vi "_PC_Daemon_SaveFiles.vi"(7 "SigProc.Enable":bool caption="SigProc", 8 "error in (no error)":errorcluster, 11 "Document Path":path) -> (0 "error out":errorcluster)   [LabVIEW 2018]
uses:
  RecipeEditorPython/subVI/getScriptInfo.ctl
  RT/PublicSubVI/Ctl/_ctl_RT_ExpCondi.ctl
  SaveFile/DataTree/ctl/FMstateMachineEnum.ctl
  PublicSubVI/Class/FileManager/FM/ctl/_PC_Pub_FM ctrlFileRefnumEnum.ctl
  PublicSubVI/Ctl/RegistyFunc.ctl
  <vilib>/Utility/miscctls.llb/LVRowAndColumnTypeDef.ctl
  <vilib>/event_ctls.llb/eventvkey.ctl
  PublicSubVI/Overload/Experiment Condition/_PC_Pub_ExpCondiValue_Script.vi
  PublicSubVI/Class/QMH/QMH.lvclass
  SaveFile/DataTree/DataTreeCtrl.lvclass
  PublicSubVI/Class/Sig2MS/Sig2MS.lvclass
panel:
  in  "Tab Control":enum32{"Document", "File"}(tab)
  in  "Document Tree":string[](tree)=["D:\\ATI_MS_InstrumentControl_08_08_15\\MSData\\Test\\Untitled.flist"]
  in  "Undo":bool
  in  "File Tree":string[](tree)
  out "wfmGraph":waveform(sgl)[](graph)
  out "XY Graph":cluster{"X":dbl[], "Y":sgl[]}[](graph)
  in  "listDataInfo":i32(listbox)=-1
  out "Item Names":string[](array[string])
  in  "mouse state":T1(ring)
  in  "timeDomain":bool caption="Time Domain"
  in  "Cursor":bool
  out "Y :":dbl
  out "X :":dbl
  in  "MergePlots":bool
  in  "SigProc.Edit":bool
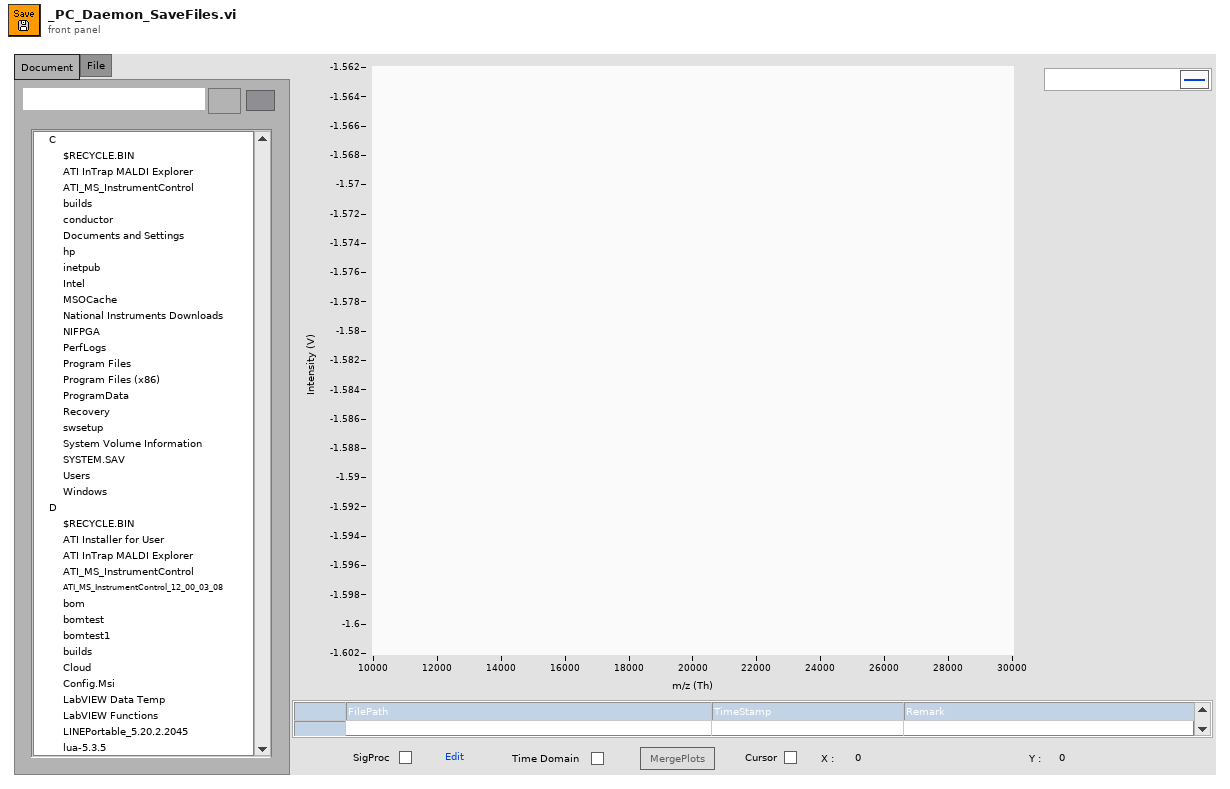
[diagram p1: front panel]
types:
  T1 = enum16{"normal", "select noise", "select signal", "return"}
  T2 = cluster{"xyGraph":refnum<vi>, "wfmGraph":refnum<vi>, "docPath in":refnum<vi>}
  T3 = enum8{"Enabled", "Disabled", "Disabled and Grayed Out"}
  T4 = cluster{"xyGraph":refnum<vi>, "wfmGraph":refnum<vi>}
  T5 = typedef "getScriptInfo.ctl" = enum16{"userEditor", "userParam", "instrParam", "sourcePath", "sourceTimeStamp", "versionInfo"}
  T6 = typedef "_ctl_RT_ExpCondi.ctl" = cluster{"Label":string, "Value":variant}[]
  T7 = cluster{"selectDataArr":string[], "tagFilePath":string}
  T8 = typedef "FMstateMachineEnum.ctl" = enum16{"none", "init", "openTDMS", "closeTDMS", "getDataList", "getDataInfo", "getTimeStamp", "getCurrPath", "getRemark", "overwriteRemark", "readData", "deleteData", "moveData"}
  T9 = typedef "_PC_Pub_FM ctrlFileRefnumEnum.ctl" = enum16{"init", "checkFileName", "updFileName", "updWorkFolder", "updDataItems", "addNewFileName", "addSerialNum"}
  T10 = cluster{"xyXLabel":string, "xyYLabel":string, "wfmXLabel":string, "wfmYLabel":string}
  T11 = cluster{"dt":dbl, "xdata":dbl[], "ydata":sgl[], "beta":dbl[]}[][]
  T12 = cluster{"startTime":dbl, "scanData":cluster{"dt":dbl, "xdata":dbl[], "ydata":sgl[], "beta":dbl[]}[], "xyXLabel":string, "xyYLabel":string, "wfmXLabel":string, "wfmYLabel":string, "ionData":cluster{"dt":dbl, "ydata":sgl[]}[], "ionXLabel":string, "ionYLabel":string}
  T13 = typedef "RegistyFunc.ctl" = enum16{"None", "FileAutoSave", "FileNoise", "FileSN", "ExeStatu", "WorkFolderPath", "MethodPath", "AVGItem", "LoopItem", "AutoRun", "BGColor", "LineColor", "LineWidth", "XGrid", "YGrid", "DeviceRefnum"}
  T14 = enum16{"init", "loadScript", "newScript", "runScript", "close"}
  T15 = typedef "LVRowAndColumnTypeDef.ctl" = cluster{"Row":i32, "Column":i32}
  T16 = typedef "eventvkey.ctl" = enum16{"ASCII", "Enter", "Return", "Shift", "Ctrl", "Alt", "Cmd", "Opt", "Caps", "NumLock", "Clear", "Break", "Up", "Down", "Left", "Right", "Insert", "Delete", "Home", "End", "PageUp", "PageDown", "Escape", "Help", "Pause", "ScrollLock", "F1", "F2", "F3", "F4", "F5", "F6", "F7", "F8", "F9", "F10", "F11", "F12", "F13", "F14", "F15", "F16", "F17", "F18", "F19", "F20", "F21", "F22", "F23", "F24", "Play", "VolumeUp", "VolumeDown", "Mute", "Two Byte Char"}
  T17 = typedef "LVPoint32TypeDef.ctl" = cluster{"Horizontal":i32, "Vertical":i32}
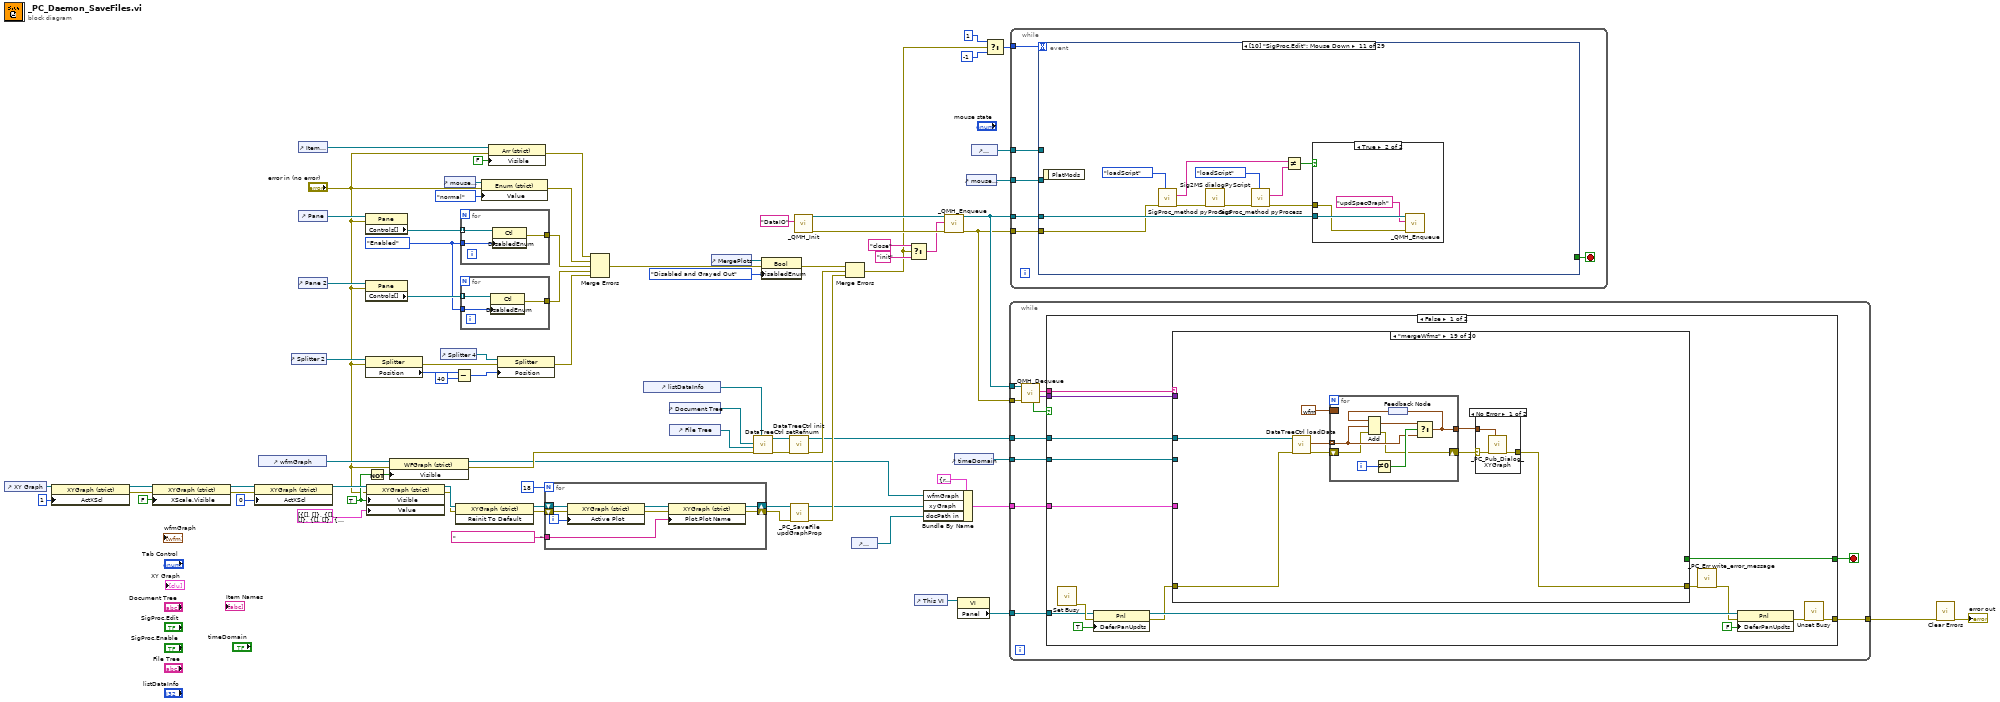
[diagram p0: block diagram]
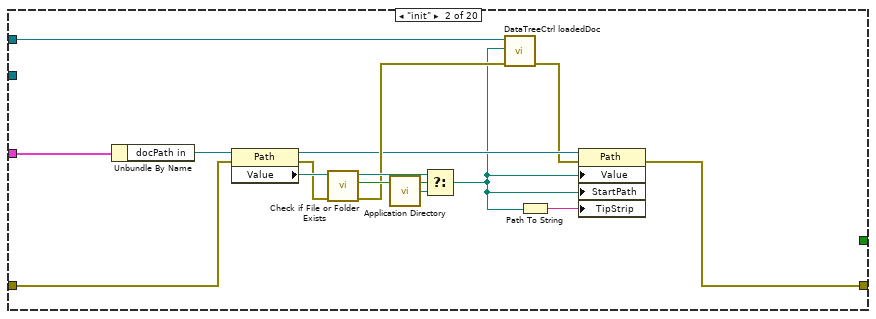
[diagram p3: hidden frame]
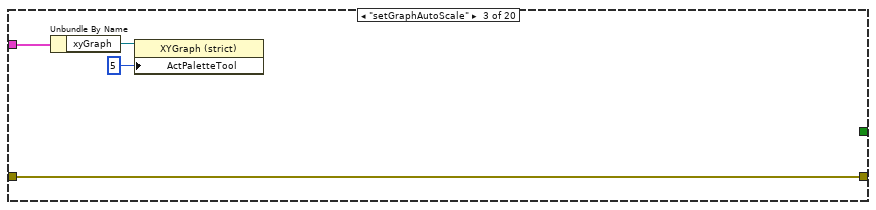
[diagram p4: hidden frame]
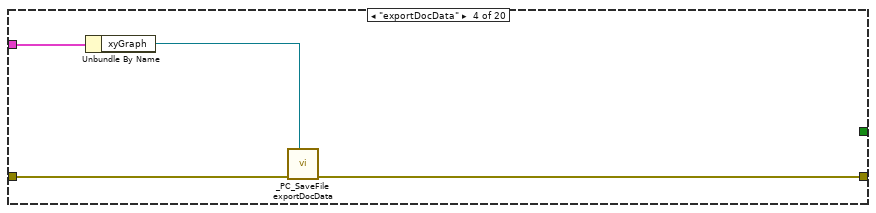
[diagram p5: hidden frame]
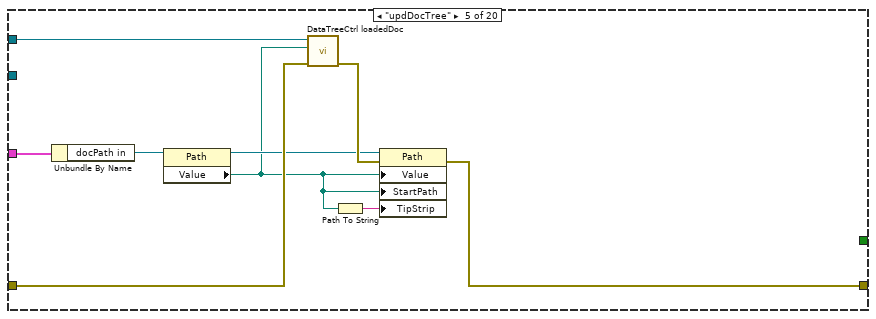
[diagram p6: hidden frame]
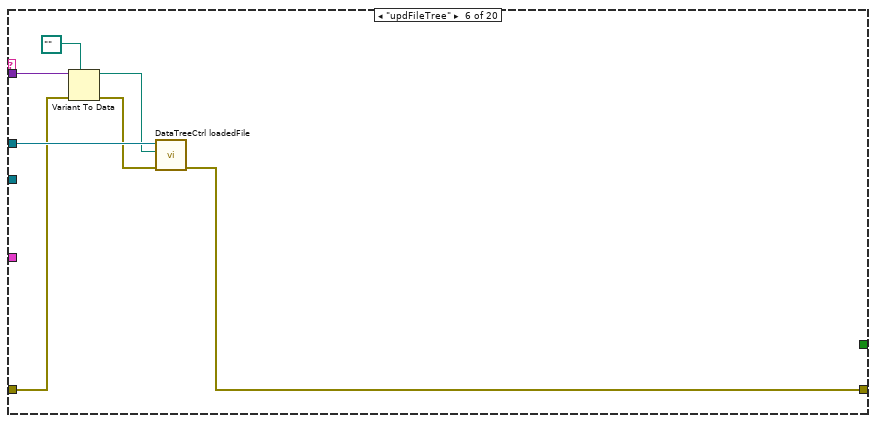
[diagram p7: hidden frame]
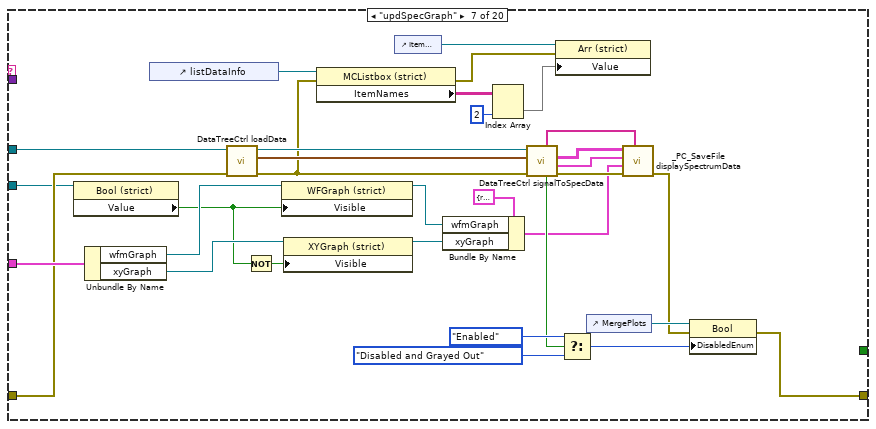
[diagram p8: hidden frame]
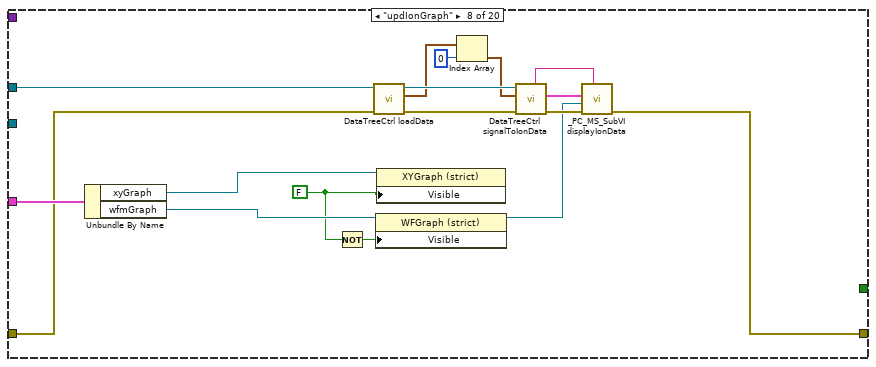
[diagram p9: hidden frame]
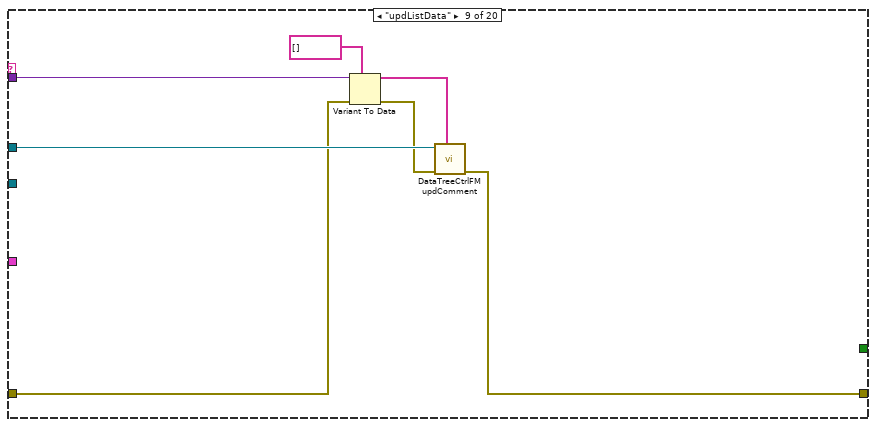
[diagram p10: hidden frame]
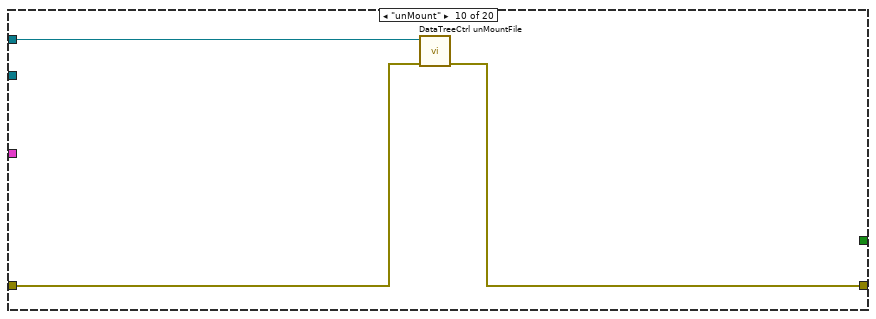
[diagram p11: hidden frame]
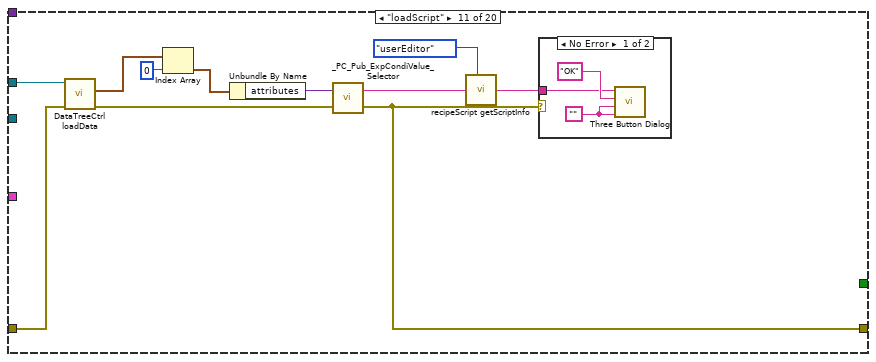
[diagram p12: hidden frame]
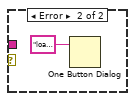
[diagram p13: hidden frame]
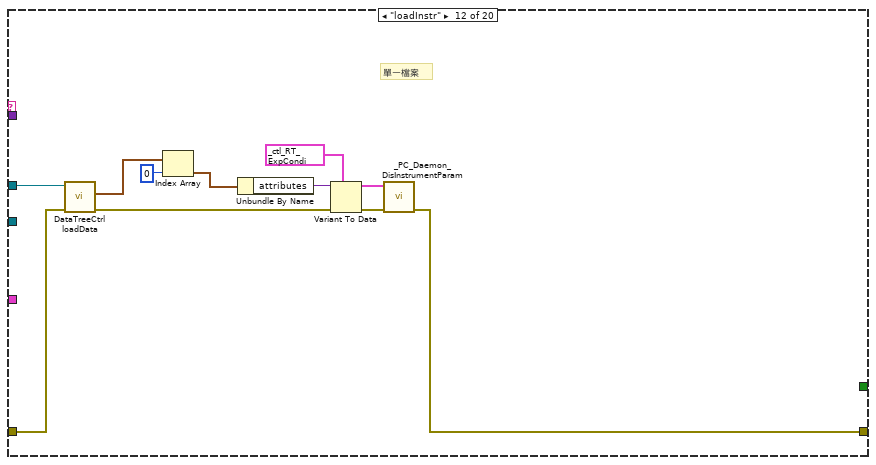
[diagram p14: hidden frame]
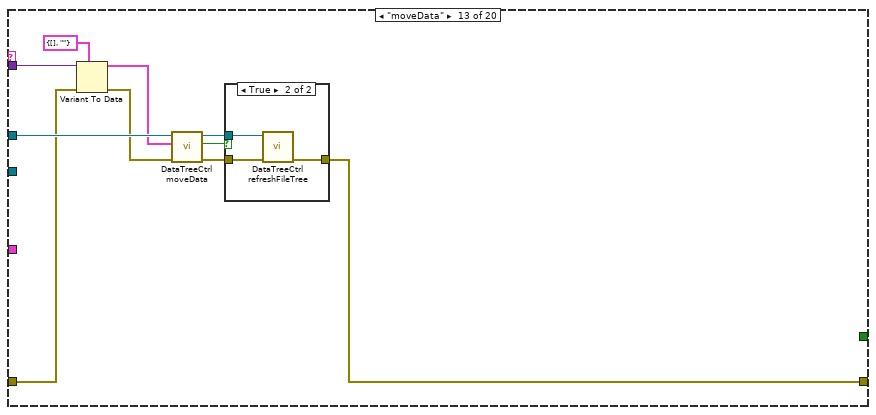
[diagram p15: hidden frame]
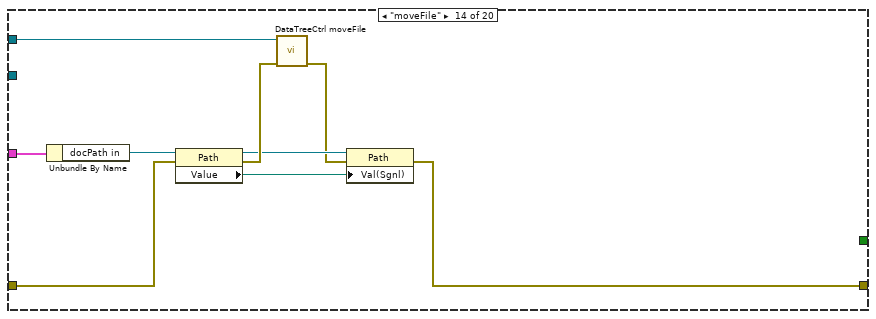
[diagram p17: hidden frame]
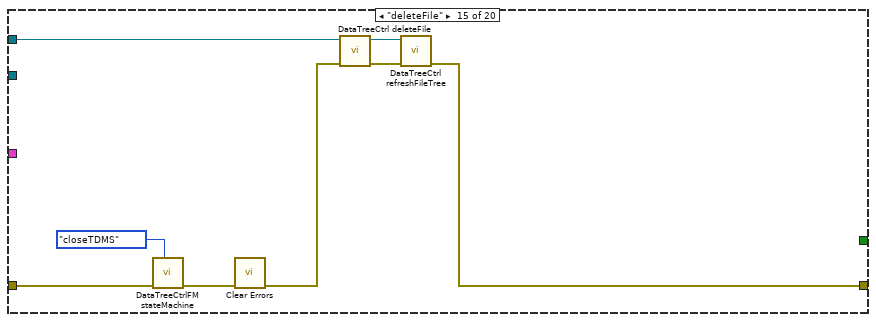
[diagram p18: hidden frame]
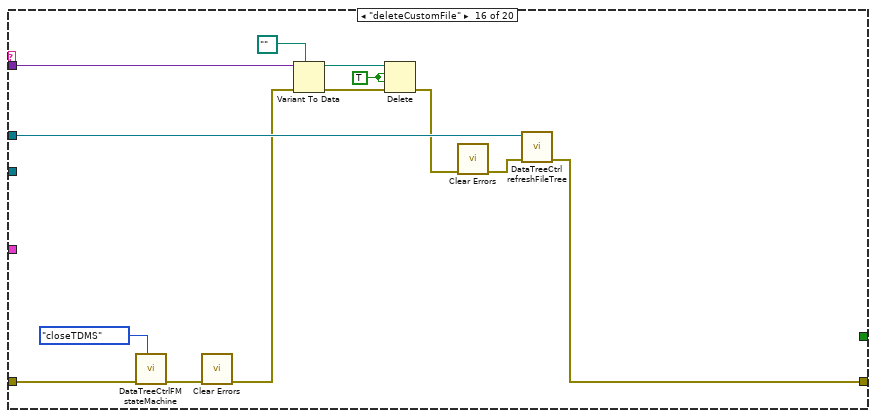
[diagram p19: hidden frame]
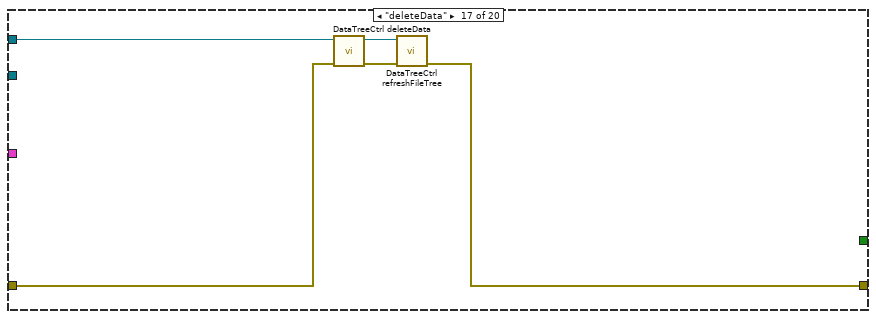
[diagram p20: hidden frame]
diagram:
  w23 = TRUE ("Visible")
  w66 = T3."Enabled" ("Disabled")
  n1 = control-ref of="XY Graph"() -> (w30:refnum<vi>)
  n2 = property class="XYGraph (strict)"(reference=w30, "ActXScl"=1 ("Active X Scale")) -> (reference out=w33:refnum<vi>, error out=w34:errorcluster)  [unwired: 1 in]
  n3 = property class="XYGraph (strict)"(reference=w33, error in=w34, "XScale.Visible"=FALSE ("X Scale.Visible")) -> (reference out=w29:refnum<vi>, error out=w28:errorcluster)
  n4 = property class="XYGraph (strict)"(reference=w29, error in=w28, "ActXScl"=0 ("Active X Scale")) -> (reference out=w26:refnum<vi>)  [unwired: 1 out]
  n5 = control-ref of="wfmGraph"() -> (w24:refnum<vi>)
  n6 = control-ref of="Splitter 2"() -> (w10:refnum<vi>)
  n7 = control-ref of="Item Names"() -> (w13:refnum<vi>)
  n8 = control-ref of="Pane"() -> (w65:refnum<vi>)
  n9 = control-ref of="Pane 2"() -> (w64:refnum<vi>)
  n10 = property class="Pane"(reference=w65, error in="error in (no error)") -> ("Controls[]"=w68:refnum<vi>[])  [unwired: 2 out]
  n11 = property class="Pane"(reference=w64, error in="error in (no error)") -> ("Controls[]"=w67:refnum<vi>[])  [unwired: 2 out]
  n12 = property class="Splitter"(reference=w10, error in="error in (no error)") -> (error out=w5:errorcluster, "Position"=w8:i32)  [unwired: 1 out]
  n13 = property class="XYGraph (strict)"(reference=w26, error in="error in (no error)", "Visible"=w23, "Value"=cluster{dbl[], sgl[]}[] [{[], []}, {[], []}, {[], []}, {[], []}, {[], []}, {[], []}, {[], []}, {[], []}, {[], []}, {[], []}, {[], []}, {[], []}, {[], []}, {[], []}, {[], []}, {[], []}, {[], []}, {[], []}] ("massSpec")) -> (reference out=w59:refnum<vi>, error out=w58:errorcluster)
  n14 = Not(x=w23) -> (.not. x?=w22:bool)
  n15 = property class="WFGraph (strict)"(reference=w24, error in="error in (no error)", "Visible"=w22) -> (reference out=w20:refnum<vi>, error out=w25:errorcluster)
  n16 = control-ref of="Splitter 4"() -> (w9:refnum<vi>)
  n17 = control-ref of="mouse state"() -> (w61:refnum<vi>)
  n18 = Subtract(x=w8, y=40) -> (x-y=w6:i32)
  n19 = invoke class="XYGraph (strict)" method="Reinit To Default"(reference=w59, error in=w58) -> (reference out=w77:refnum<vi>, error out=w52:errorcluster)  [unwired: 1 in, 1 out]
  n20 = for {
    tunnel: w68 -> [w82] mode=indexing
    tunnel: w66 -> [w81]
    tunnel: [w80] -> w63
    n21 = property class="Ctl"(reference=w82, "DisabledEnum"=w81) -> (error out=w80:errorcluster)  [unwired: 1 in, 1 out]
  }
  n22 = for {
    tunnel: w67 -> [w85] mode=indexing
    tunnel: w66 -> [w84]
    tunnel: [w83] -> w62
    n23 = property class="Ctl"(reference=w85, "DisabledEnum"=w84) -> (error out=w83:errorcluster)  [unwired: 1 in, 1 out]
  }
  n24 = property class="Enum (strict)"(reference=w61, error in="error in (no error)", "Value"=T1."normal") -> (error out=w60:errorcluster)  [unwired: 1 out]
  n25 = property class="Arr (strict)"(reference=w13, error in="error in (no error)", "Visible"=FALSE) -> (error out=w11:errorcluster)  [unwired: 1 out]
  n26 = property class="Splitter"(reference=w9, error in=w5, "Position"=w6) -> (error out=w3:errorcluster)  [unwired: 1 out]
  n27 = for {
    N: 18 -> [_]
    tunnel: "                                          " -> [w91]
    shift-right: [w86] -> w51
    shift-left: w52 -> [w87]
    shift-right: [w88] -> w72
    shift-left: w77 -> [w93]
    i -> [w92]
    n28 = property class="XYGraph (strict)"(reference=w93, error in=w87, "Active Plot"=w92) -> (reference out=w90:refnum<vi>, error out=w89:errorcluster)
    n29 = property class="XYGraph (strict)"(reference=w90, error in=w89, "Plot.Plot Name"=w91) -> (reference out=w88:refnum<vi>, error out=w86:errorcluster)
  }
  n30 = Merge Errors(w11, w60, w63, w62, w3) -> (w2:errorcluster)
  n31 = control-ref of="listDataInfo"() -> (w14:refnum<vi>)
  n32 = control-ref of="Document Tree"() -> (w56:refnum<vi>)
  n33 = control-ref of="File Tree"() -> (w55:refnum<vi>)
  n34 = control-ref of="MergePlots"() -> (w71:refnum<vi>)
  n35 = call "DataTreeCtrl setRefnum.vi"("listDataInfo"=w14, "error in (no error)"=w25, "File Tree"=w55, "Document Tree"=w56) -> ("error out"=w53:errorcluster, "DataTreeCtrl out"=w54:refnum<class "DataTreeCtrl.lvclass">)  [unwired: 6 in]
  n36 = property class="Bool"(reference=w71, error in=w2, "DisabledEnum"=T3."Disabled and Grayed Out" ("Disabled")) -> (error out=w50:errorcluster)  [unwired: 1 out]
  n37 = call "DataTreeCtrl init.vi"("error in (no error)"=w53, "DataTreeCtrl in"=w54) -> ("error out"=w49:errorcluster, "DataTreeCtrl out"=w41:refnum<class "DataTreeCtrl.lvclass">)  [unwired: 8 in]
  n38 = call "_PC_SaveFile updGraphProp.vi"("error in (no error)"=w51, "XY Graph in"=w72) -> ("error out"=w48:errorcluster, "XY Graph out"=w44:refnum<vi>)  [unwired: 8 in]
  n39 = call "_QMH_Init.vi"("name (unnamed)"="DataIO") -> ("error out"=w73:errorcluster, "QMH out"=w74:refnum<class "QMH.lvclass">)  [unwired: 9 in]
  n40 = Merge Errors(w50, w49, w48) -> (w1:errorcluster)
  n41 = control-ref of="Document Path"() -> (w43:refnum<vi>)
  n42 = Select(t="close" ("Msg"), s=w1, f="init" ("Msg")) -> (s? t:f=w45:string)
  n43 = control-ref of="This VI"() -> (w78:refnum<vi>)
  n44 = Bundle By Name(cluster=T2 {"xyGraph"=refnum, "wfmGraph"=refnum, "docPath in"=refnum}, "wfmGraph"=w20, "xyGraph"=w44, "docPath in"=w43) -> (w42:T2)
  n45 = call "_QMH_Enqueue.vi"("error in (no error)"=w73, "Msg"=w45, "QMH in"=w74) -> ("error out"=w39:errorcluster, "QMH out"=w40:refnum<class "QMH.lvclass">)  [unwired: 7 in]
  n46 = control-ref of="timeDomain"() -> (w19:refnum<vi>)
  n47 = property class="VI"(reference=w78) -> ("Panel"=w38:refnum<vi>)  [unwired: 1 in, 2 out]
  n48 = control-ref of="mouse state"() -> (w69:refnum<vi>)
  n49 = control-ref of="Document Path"() -> (w37:refnum<vi>)
  n50 = Select(t=1, s=w1, f=-1) -> (s? t:f=w15:i32)
  n51 = while {
    tunnel: w42 -> [w98]
    tunnel: w41 -> [w97]
    tunnel: w40 -> [w104]
    tunnel: w39 -> [w103]
    tunnel: w38 -> [w99]
    tunnel: [w95] -> w36
    tunnel: w19 -> [w94]
    stop <- w96 stop-if-true
    n52 = call "_QMH_Dequeue.vi"("error in (no error)"=w103, "QMH in"=w104) -> ("Data"=w100:variant, "Msg"=w101:string, "timed out?"=w102:bool)  [unwired: 4 in, 3 out]
    n53 = case shown="False" w102 {
      tunnel: w101 -> [w120 _]
      tunnel: w100 -> [w119 _]
      tunnel: w99 -> [w116 _]
      tunnel: w98 -> [w109 _]
      tunnel: w97 -> [w108 _]
      tunnel: [w107 _] -> w96
      tunnel: [w106 _] -> w95
      tunnel: w94 -> [w105 _]
      frame False {
        n54 = call <vilib>:"Set Busy.vi"() -> ("error out"=w117:errorcluster)  [unwired: 10 in, 1 out]
        n55 = property class="Pnl"(reference=w116, error in=w117, "DeferPanUpdts"=TRUE ("Defer Panel Updates")) -> (reference out=w113:refnum<vi>, error out=w110:errorcluster)
        n56 = case shown="\"mergeWfms\"" w120 {
          tunnel: w119 -> [_ _ _ _ _ w159 _ _ w214 _ _ _ w251 _ _ w288 _ _ _ _]
          tunnel: [w121 w134 w137 w141 w145 w154 w186 w199 w215 w217 w224 w235 w246 w260 w271 w289 w290 w295 w300 w322] -> w111
          tunnel: w110 -> [w121 w122 w137 w142 w148 w156 w182 w207 w212 w218 w223 w241 w248 w265 w272 w279 w293 w296 w304 w319]
          tunnel: w109 -> [_ w135 w139 w144 w152 _ w192 w209 _ _ _ _ _ w267 _ _ _ _ _ _]
          tunnel: w108 -> [_ w136 _ _ w153 w160 w191 w208 w216 w219 w230 w245 w252 w268 w276 w283 w294 w297 w305 _]
          tunnel: [_ _ _ _ _ _ _ _ _ _ _ _ _ _ _ _ _ _ _ TRUE] -> w107
          tunnel: w105 -> [_ _ _ _ _ _ w176 _ _ _ _ _ _ _ _ _ _ _ _ _]
          frame Default {
          }
          frame "init" {
            n57 = Unbundle By Name(w135) -> ("docPath in"=w130:refnum<vi>)
            n58 = property class="Path"(reference=w130, error in=w122) -> (reference out=w126:refnum<vi>, error out=w128:errorcluster, "Value"=w129:path)
            n59 = call <vilib>:"Check if File or Folder Exists.vi"("error in (no error)"=w128, "path"=w129) -> ("error out"=w127:errorcluster, "file or folder exists?"=w133:bool, "dup path"=w132:path)  [unwired: 7 in]
            n60 = call <vilib>:"Application Directory.vi"() -> ("Application Directory"=w131:path)
            n61 = Select(t=w132, s=w133, f=w131) -> (s? t:f=w125:path)
            n62 = call "DataTreeCtrl loadedDoc.vi"("error in (no error)"=w127, "RootPath"=w125, "DataTreeCtrl in"=w136) -> ("error out"=w123:errorcluster)  [unwired: 7 in, 1 out]
            n63 = Path To String(path=w125) -> (string=w124:string)
            n64 = property class="Path"(reference=w126, error in=w123, "Value"=w125, "StartPath"=w125, "TipStrip"=w124) -> (error out=w134:errorcluster)  [unwired: 1 out]
          }
          frame "setGraphAutoScale" {
            n65 = Unbundle By Name(w139) -> ("xyGraph"=w138:refnum<vi>)
            n66 = property class="XYGraph (strict)"(reference=w138, "ActPaletteTool"=5 ("Palette:Active Tool")) -> ()  [unwired: 1 in, 2 out]
          }
          frame "exportDocData" {
            n67 = Unbundle By Name(w144) -> ("xyGraph"=w143:refnum<vi>)
            n68 = call "_PC_SaveFile exportDocData.vi"("xy graph ref"=w143, "error in (no error)"=w142) -> ("error out"=w141:errorcluster)  [unwired: 9 in]
          }
          frame "updDocTree" {
            n69 = Unbundle By Name(w152) -> ("docPath in"=w149:refnum<vi>)
            n70 = property class="Path"(reference=w149) -> (reference out=w147:refnum<vi>, "Value"=w146:path)  [unwired: 1 in, 1 out]
            n71 = call "DataTreeCtrl loadedDoc.vi"("error in (no error)"=w148, "RootPath"=w146, "DataTreeCtrl in"=w153) -> ("error out"=w151:errorcluster)  [unwired: 7 in, 1 out]
            n72 = Path To String(path=w146) -> (string=w150:string)
            n73 = property class="Path"(reference=w147, error in=w151, "Value"=w146, "StartPath"=w146, "TipStrip"=w150) -> (error out=w145:errorcluster)  [unwired: 1 out]
          }
          frame "updFileTree" {
            n74 = Variant To Data(error in=w156, type=path "", Variant=w159) -> (data=w157:path, error out=w155:errorcluster)
            n75 = call "DataTreeCtrl loadedFile.vi"("error in (no error)"=w155, "filePath"=w157, "DataTreeCtrl in"=w160) -> ("error out"=w154:errorcluster)  [unwired: 7 in, 1 out]
          }
          frame "updSpecGraph" {
            n76 = property class="Bool (strict)"(reference=w176) -> ("Value"=w172:bool)  [unwired: 1 in, 2 out]
            n77 = Unbundle By Name(w192) -> ("wfmGraph"=w175:refnum<vi>, "xyGraph"=w173:refnum<vi>)
            n78 = control-ref of="listDataInfo"() -> (w162:refnum<vi>)
            n79 = call "DataTreeCtrl loadData.vi"("error in (no error)"=w182, "DataTreeCtrl in"=w191) -> ("error out"=w161:errorcluster, "signalMultiData"=w184:waveform(sgl)[], "DataTreeCtrl out"=w185:refnum<class "DataTreeCtrl.lvclass">)  [unwired: 7 in]
            n80 = Not(x=w172) -> (.not. x?=w171:bool)
            n81 = property class="WFGraph (strict)"(reference=w175, "Visible"=w172) -> (reference out=w174:refnum<vi>)  [unwired: 1 in, 1 out]
            n82 = property class="XYGraph (strict)"(reference=w173, "Visible"=w171) -> (reference out=w170:refnum<vi>)  [unwired: 1 in, 1 out]
            n83 = property class="MCListbox (strict)"(reference=w162, error in=w161) -> (error out=w166:errorcluster, "ItemNames"=w164:string[][])  [unwired: 1 out]
            n84 = control-ref of="Item Names"() -> (w167:refnum<vi>)
            n85 = Bundle By Name(cluster=T4 {"xyGraph"=refnum, "wfmGraph"=refnum} ("graphRefnum in"), "wfmGraph"=w174, "xyGraph"=w170) -> (w178:T4)
            n86 = Index Array(array=w164, index (col)=2 ("disabled index (col)")) -> (element=w163:string[])  [unwired: 1 in]
            n87 = call "DataTreeCtrl signalToSpecData.vi"("error in (no error)"=w161, "signalMultiData"=w184, "DataTreeCtrl in"=w185) -> ("error out"=w180:errorcluster, "labelName"=w169:T10, "scanSigInfo"=w168:T11, "mergeValid?"=w183:bool, "plotName"=w181:string[])  [unwired: 3 in, 1 out]
            n88 = property class="Arr (strict)"(reference=w167, error in=w166, "Value"=w163) -> ()  [unwired: 2 out]
            n89 = Select(t=T3."Enabled" ("Disabled"), s=w183, f=T3."Disabled and Grayed Out") -> (s? t:f=w187:T3)
            n90 = control-ref of="MergePlots"() -> (w190:refnum<vi>)
            n91 = call "_PC_SaveFile displaySpectrumData.vi"("plotNameArr"=w181, "error in (no error)"=w180, "graphRefnum in"=w178, "labelName"=w169, "newScanData"=w168) -> ("error out"=w179:errorcluster)  [unwired: 5 in, 1 out]
            n92 = property class="Bool"(reference=w190, error in=w179, "DisabledEnum"=w187) -> (error out=w186:errorcluster)  [unwired: 1 out]
          }
          frame "updIonGraph" {
            w195 = FALSE
            n93 = Unbundle By Name(w209) -> ("xyGraph"=w198:refnum<vi>, "wfmGraph"=w197:refnum<vi>)
            n94 = Not(x=w195) -> (.not. x?=w194:bool)
            n95 = call "DataTreeCtrl loadData.vi"("error in (no error)"=w207, "DataTreeCtrl in"=w208) -> ("error out"=w202:errorcluster, "signalMultiData"=w205:waveform(sgl)[], "DataTreeCtrl out"=w206:refnum<class "DataTreeCtrl.lvclass">)  [unwired: 7 in]
            n96 = property class="WFGraph (strict)"(reference=w197, "Visible"=w194) -> (reference out=w196:refnum<vi>)  [unwired: 1 in, 1 out]
            n97 = property class="XYGraph (strict)"(reference=w198, "Visible"=w195) -> ()  [unwired: 1 in, 2 out]
            n98 = Index Array(array=w205, index=0) -> (element=w203:waveform(sgl))
            n99 = call "DataTreeCtrl signalToIonData.vi"("error in (no error)"=w202, "signalData"=w203, "DataTreeCtrl in"=w206) -> ("error out"=w201:errorcluster, "ionSigInfo"=w193:T12, "plotName"=w200:string)  [unwired: 5 in, 1 out]
            n100 = call "_PC_MS_SubVI displayIonData.vi"("plotName"=w200, "error in (no error)"=w201, "wfmGraph"=w196, "ionSigInfo"=w193) -> ("error out"=w199:errorcluster)  [unwired: 7 in]
          }
          frame "updListData" {
            n101 = Variant To Data(error in=w212, type=string[] [] ("Value"), Variant=w214) -> (data=w210:string[], error out=w211:errorcluster)
            n102 = call "DataTreeCtrlFM updComment.vi"("newItemNames"=w210, "error in (no error)"=w211, "DataTreeCtrl in"=w216) -> ("error out"=w215:errorcluster)  [unwired: 7 in, 1 out]
          }
          frame "unMount" {
            n103 = call "DataTreeCtrl unMountFile.vi"("error in (no error)"=w218, "DataTreeCtrl in"=w219) -> ("error out"=w217:errorcluster)  [unwired: 8 in, 1 out]
          }
          frame "loadScript" {
            n104 = call "DataTreeCtrl loadData.vi"("error in (no error)"=w223, "DataTreeCtrl in"=w230) -> ("error out"=w227:errorcluster, "signalMultiData"=w229:waveform(sgl)[])  [unwired: 7 in, 1 out]
            n105 = Index Array(array=w229, index=0) -> (element=w226:waveform(sgl))
            n106 = Unbundle By Name(w226) -> ("attributes"=w225:variant)
            n107 = call-poly "_PC_Pub_ExpCondiValue_Selector.vi"("error in (no error)"=w227, "expCondiVariant"=w225) -> ("error out"=w224:errorcluster, "scriptCode"=w222:string)
            n108 = call "recipeScript getScriptInfo.vi"("sysCode"=w222, "method"=getScriptInfo."userEditor") -> ("output"=w221:string)  [unwired: 1 in]
            n109 = case shown="No Error" w224 {
              tunnel: w221 -> [w231 _]
              frame No Error {
                w233 = ""
                n110 = call <vilib>:"Three Button Dialog.vi"("Right Button Text (\"Cancel\")"=w233, "Center Button Text (\"No\")"=w233, "Left Button Text (\"Yes\")"="OK" ("Left Button Text (\"Yes\")"), "message"=w231) -> ()  [unwired: 7 in, 1 out]
              }
              frame Error {
                n111 = One Button Dialog(message="load script failure") -> ()  [unwired: 1 in, 1 out]
              }
            }
          }
          frame "loadInstr" {
            # "單一檔案"
            n112 = call "DataTreeCtrl loadData.vi"("error in (no error)"=w241, "DataTreeCtrl in"=w245) -> ("error out"=w238:errorcluster, "signalMultiData"=w244:waveform(sgl)[])  [unwired: 7 in, 1 out]
            n113 = Index Array(array=w244, index=0) -> (element=w242:waveform(sgl))
            n114 = Unbundle By Name(w242) -> ("attributes"=w239:variant)
            n115 = Variant To Data(error in=w238, type=T6 [{"Label"="Laser", "Value"=variant}, {"Label"="Pressure", "Value"=variant}, {"Label"="TMP", "Value"=variant}, {"Label"="Script", "Value"=variant}, {"Label"="Signal Remarks", "Value"=variant}, {"Label"="ExtAO", "Value"=variant}, {"Label"="ExtDO", "Value"=variant}, {"Label"="ExtDI", "Value"=variant}, {"Label"="D999", "Value"=variant}] ("ExpCondi"), Variant=w239) -> (data=w237:T6, error out=w236:errorcluster)
            n116 = call "_PC_Daemon_DisInstrumentParam.vi"("error in"=w236, "ExpCondi"=w237) -> ("error out"=w235:errorcluster)  [unwired: 9 in]
          }
          frame "moveData" {
            n117 = Variant To Data(error in=w248, type=T7 {"selectDataArr"=[], "tagFilePath"=""}, Variant=w251) -> (data=w249:T7, error out=w247:errorcluster)
            n118 = call "DataTreeCtrl moveData.vi"("error in (no error)"=w247, "moveParam"=w249, "DataTreeCtrl in"=w252) -> ("error out"=w254:errorcluster, "accepted"=w253:bool, "DataTreeCtrl out"=w255:refnum<class "DataTreeCtrl.lvclass">)  [unwired: 6 in]
            n119 = case shown="True" w253 {
              tunnel: w255 -> [_ w259]
              tunnel: w254 -> [w256 w258]
              tunnel: [w256 w257] -> w246
              frame False {
              }
              frame True {
                n120 = call "DataTreeCtrl refreshFileTree.vi"("error in (no error)"=w258, "DataTreeCtrl in"=w259) -> ("error out"=w257:errorcluster)  [unwired: 8 in, 1 out]
              }
            }
          }
          frame "moveFile" {
            n121 = Unbundle By Name(w267) -> ("docPath in"=w266:refnum<vi>)
            n122 = property class="Path"(reference=w266, error in=w265) -> (reference out=w263:refnum<vi>, error out=w264:errorcluster, "Value"=w261:path)
            n123 = call "DataTreeCtrl moveFile.vi"("error in (no error)"=w264, "DataTreeCtrl in"=w268) -> ("error out"=w262:errorcluster)  [unwired: 8 in, 1 out]
            n124 = property class="Path"(reference=w263, error in=w262, "Val(Sgnl)"=w261) -> (error out=w260:errorcluster)  [unwired: 1 out]
          }
          frame "deleteFile" {
            n125 = call "DataTreeCtrlFM stateMachine.vi"("Func"=FMstateMachineEnum."closeTDMS", "error in (no error)"=w272) -> ("error out"=w270:errorcluster)  [unwired: 4 in, 5 out]
            n126 = call <vilib>:"Clear Errors.vi"("error in (no error)"=w270) -> ("error out"=w269:errorcluster)  [unwired: 5 in, 1 out]
            n127 = call "DataTreeCtrl deleteFile.vi"("error in (no error)"=w269, "DataTreeCtrl in"=w276) -> ("error out"=w274:errorcluster, "DataTreeCtrl out"=w275:refnum<class "DataTreeCtrl.lvclass">)  [unwired: 8 in]
            n128 = call "DataTreeCtrl refreshFileTree.vi"("error in (no error)"=w274, "DataTreeCtrl in"=w275) -> ("error out"=w271:errorcluster)  [unwired: 8 in, 1 out]
          }
          frame "deleteCustomFile" {
            w286 = TRUE ("confirm (F)")
            n129 = call "DataTreeCtrlFM stateMachine.vi"("Func"=FMstateMachineEnum."closeTDMS", "error in (no error)"=w279) -> ("error out"=w278:errorcluster)  [unwired: 4 in, 5 out]
            n130 = call <vilib>:"Clear Errors.vi"("error in (no error)"=w278) -> ("error out"=w277:errorcluster)  [unwired: 5 in, 1 out]
            n131 = Variant To Data(error in=w277, type=path "" ("path"), Variant=w288) -> (data=w285:path, error out=w284:errorcluster)
            n132 = Delete(path (use dialog)=w285, entire hierarchy (F)=w286, confirm (F)=w286, error in=w284) -> (error out=w282:errorcluster)  [unwired: 1 in, 2 out]
            n133 = call <vilib>:"Clear Errors.vi"("error in (no error)"=w282) -> ("error out"=w281:errorcluster)  [unwired: 5 in, 1 out]
            n134 = call "DataTreeCtrl refreshFileTree.vi"("error in (no error)"=w281, "DataTreeCtrl in"=w283) -> ("error out"=w289:errorcluster)  [unwired: 8 in, 1 out]
          }
          frame "deleteData" {
            n135 = call "DataTreeCtrl deleteData.vi"("error in (no error)"=w293, "DataTreeCtrl in"=w294) -> ("error out"=w292:errorcluster, "DataTreeCtrl out"=w291:refnum<class "DataTreeCtrl.lvclass">)  [unwired: 8 in]
            n136 = call "DataTreeCtrl refreshFileTree.vi"("error in (no error)"=w292, "DataTreeCtrl in"=w291) -> ("error out"=w290:errorcluster)  [unwired: 8 in, 1 out]
          }
          frame "saveAsMAT" {
            n137 = call "DataTreeCtrl saveAsMAT.vi"("error in (no error)"=w296, "DataTreeCtrl in"=w297) -> ("error out"=w295:errorcluster)  [unwired: 8 in, 1 out]
          }
          frame "mergeWfms" {
            n138 = call "DataTreeCtrl loadData.vi"("error in (no error)"=w304, "DataTreeCtrl in"=w305) -> ("error out"=w302:errorcluster, "signalMultiData"=w303:waveform(sgl)[])  [unwired: 7 in, 1 out]
            n139 = for {
              tunnel: [w315] -> w298
              tunnel: w303 -> [w312] mode=indexing
              shift-right: [w310] -> w299
              shift-left: w302 -> [w311]
              border: waveform(sgl) {"t0"=timestamp(0 s since 1904-01-01), "dt"=1.0, "Y"=[]} ("signalData") -> [_]
              i -> [w317]
              n140 = Not Equal To 0?(x=w317) -> (x != 0?=w316:bool)
              n141 = feedback #1() -> (w313:waveform(sgl))
              n142 = Add(1:w312, 2:w313, 4:w311) -> (0:w314:waveform(sgl), 3:w310:errorcluster)
              n143 = Select(t=w314, s=w316, f=w312) -> (s? t:f=w315:waveform(sgl))
              n144 = feedback-in #1(w315) -> ()
            }
            n145 = case shown="No Error" w299 {
              selector: w299 -> [w308 w309]
              tunnel: [w307 w309] -> w300
              tunnel: w298 -> [w306 _]
              frame No Error {
                n146 = call "_PC_Pub_Dialog_XYGraph.vi"("signal in"=w306, "error in (no error)"=w308) -> ("error out"=w307:errorcluster)  [unwired: 9 in]
              }
              frame Error {
              }
            }
          }
          frame "close" {
            n147 = call "DataTreeCtrlFM stateMachine.vi"("Func"=FMstateMachineEnum."closeTDMS", "error in (no error)"=w319) -> ("error out"=w318:errorcluster)  [unwired: 4 in, 5 out]
            n148 = call <vilib>:"Clear Errors.vi"("error in (no error)"=w318) -> ("error out"=w321:errorcluster)  [unwired: 5 in, 1 out]
            n149 = call "_PC_Pub_FM ctrlInstrRefNum.vi"("function"=_PC_Pub_FM_ctrlFileRefnumEnum."updDataItems", "error in (no error)"=w321) -> ("error out"=w322:errorcluster)  [unwired: 9 in]
          }
        }
        n150 = call "_PC_Err write_error_message.vi"("error in"=w111) -> ("error out"=w112:errorcluster)  [unwired: 10 in]
        n151 = property class="Pnl"(reference=w113, error in=w112, "DeferPanUpdts"=FALSE ("Defer Panel Updates")) -> (error out=w114:errorcluster)  [unwired: 1 out]
        n152 = call <vilib>:"Unset Busy.vi"("error in (no error)"=w114) -> ("error out"=w106:errorcluster)  [unwired: 10 in]
      }
      frame True {
      }
    }
  }
  n153 = while {
    tunnel: w40 -> [w330]
    tunnel: w39 -> [w329]
    tunnel: w69 -> [w327]
    tunnel: w37 -> [w326]
    tunnel: w15 -> [w325]
    stop <- w328 stop-if-true
    n154 = event shown="[10] \"SigProc.Edit\": Mouse Down" {
      selector: _ -> [_ _ _ _ _ _ _ _ _ _ _ _ _ _ _ _ _ _ _ _ _ _ _ _ _ _ _ _ _]
      dyn-events: _ -> [_ _ _ _ _ _ _ _ _ _ _ _ _ _ _ _ _ _ _ _ _ _ _ _ _ _ _ _ _]
      timeout: w325 -> [_ _ _ _ _ _ _ _ _ _ _ _ _ _ _ _ _ _ _ _ _ _ _ _ _ _ _ _ _]
      tunnel: w330 -> [_ _ w335 _ _ _ w380 _ w415 w419 w441 w446 _ w459 w480 w504 _ _ w518 w535 _ _ w622 w660 w670 _ w730 w738 w744]
      tunnel: w329 -> [_ _ w336 _ _ _ w377 _ w414 w422 w438 w445 w449 w460 w472 w494 _ _ w521 w534 _ w616 w621 w659 w669 _ w729 w737 w743]
      tunnel: [TRUE _ _ _ _ _ _ _ _ _ _ _ _ _ _ _ _ _ _ _ _ _ _ _ _ _ _ TRUE w740] -> w328
      tunnel: w327 -> [_ _ _ _ w349 w360 w385 _ _ _ _ _ _ _ _ _ _ _ _ _ _ _ _ _ _ _ _ _ _]
      tunnel: w326 -> [_ _ _ _ _ _ _ _ _ _ _ _ _ _ _ _ _ _ w516 _ _ _ _ _ _ _ _ _ _]
      event Timeout {
        n155 = event-data() -> ()  [unwired: 1 in, 3 out]
      }
      event Mouse Move {
        n156 = event-data() -> ()  [unwired: 1 in, 1 out]
        n157 = call "_PC_Pub ctrlRegistry.vi"("type"=enum16{"None", "Write", "Read"}."Write", "function"=RegistyFunc."ExeStatu", "write value"=u32 1) -> ()  [unwired: 5 in, 4 out]
      }
      event "XY Graph": Shortcut Menu Selection (User) {
        n158 = event-data() -> ("ItemTag"=w337:string)  [unwired: 1 in]
        n159 = case shown="\"exportDocData\"" w337 {
          selector: w337 -> [_ w338]
          tunnel: w336 -> [_ w339]
          tunnel: w335 -> [_ w340]
          frame Default {
          }
          frame "exportDocData" {
            n160 = call "_QMH_Enqueue.vi"("error in (no error)"=w339, "Msg"=w338, "QMH in"=w340) -> ()  [unwired: 7 in, 2 out]
          }
        }
      }
      event "XY Graph": Mouse Down? {
        w341 = u8 0 ("X Scale.Scale Fit")
        n161 = event-data() -> ("CtlRef"=w342:refnum<vi>)  [unwired: 1 in]
        n162 = property class="XYGraph (strict)"(reference=w342, "XScale.ScaleFit"=w341, "YScale.ScaleFit"=w341) -> ()  [unwired: 1 in, 2 out]
        n163 = event-data("Discard?"=FALSE) -> ()  [unwired: 1 in, 1 out]
      }
      event "XY Graph": Mouse Down {
        n164 = event-data() -> ("CtlRef"=w347:refnum<vi>, "Coords"=w346:T17)  [unwired: 1 in]
        n165 = property class="Enum (strict)"(reference=w349) -> (error out=w345:errorcluster, "Value"=w348:T1)  [unwired: 1 in, 1 out]
        n166 = case shown="\"select noise\", \"select signal\"" w348 {
          tunnel: w347 -> [_ w351]
          tunnel: w346 -> [_ w353]
          tunnel: w345 -> [_ w352]
          tunnel: enum16{"none", "down", "move", "up"}."down" ("mouse type") -> [_ w350]
          frame "normal", Default {
          }
          frame "select noise", "select signal" {
            n167 = call "_PC_Spectrafilter enable_draw_rectangle.vi"("error in (no error)"=w352, "mouse type"=w350, "Point32"=w353, "xy graph ref"=w351) -> ()  [unwired: 5 in, 3 out]
          }
        }
      }
      event "XY Graph": Mouse Move {
        n168 = event-data() -> ("CtlRef"=w358:refnum<vi>, "Coords"=w357:T17)  [unwired: 1 in]
        n169 = property class="Enum (strict)"(reference=w360) -> (error out=w356:errorcluster, "Value"=w359:T1)  [unwired: 1 in, 1 out]
        n170 = case shown="\"normal\", Default" w359 {
          tunnel: w358 -> [w363 w373]
          tunnel: w357 -> [w362 w376]
          tunnel: w356 -> [w364 w375]
          tunnel: enum16{"none", "down", "move", "up"}."move" ("mouse type") -> [_ w374]
          tunnel: "Cursor" -> [w361 _]
          frame "normal", Default {
            n171 = case shown="False" w361 {
              tunnel: w364 -> [_ w372]
              tunnel: w363 -> [_ w371]
              tunnel: w362 -> [_ w368]
              frame False {
              }
              frame True {
                n172 = invoke class="XYGraph (strict)" method="Map Coords To XY"(reference=w371, error in=w372, "Coords"=w368) -> (reference out=w370:refnum<vi>, error out=w369:errorcluster, "XY"=w367:cluster{"X":dbl, "Y":dbl})  [unwired: 4 in, 4 out]
                n173 = Unbundle By Name(w367) -> ("X"=→"X :":dbl, "Y"=→"Y :":dbl)
                n174 = property class="XYGraph (strict)"(reference=w370, error in=w369, "Cursor.Cursor Position"=w367) -> ()  [unwired: 2 out]
              }
            }
          }
          frame "select noise", "select signal" {
            n175 = call "_PC_Spectrafilter enable_draw_rectangle.vi"("error in (no error)"=w375, "mouse type"=w374, "Point32"=w376, "xy graph ref"=w373) -> ()  [unwired: 5 in, 3 out]
          }
        }
      }
      event "XY Graph": Mouse Up {
        n176 = event-data() -> ("CtlRef"=w383:refnum<vi>, "Coords"=w382:T17)  [unwired: 1 in]
        n177 = property class="Enum (strict)"(reference=w385, error in=w377) -> (reference out=w379:refnum<vi>, error out=w381:errorcluster, "Value"=w384:T1)
        n178 = case shown="\"select signal\"" w384 {
          tunnel: w383 -> [_ w390 w403]
          tunnel: w382 -> [_ w389 w402]
          tunnel: w381 -> [_ w392 w405]
          tunnel: w380 -> [_ w395 w406]
          tunnel: w379 -> [_ _ _]
          tunnel: enum16{"none", "down", "move", "up"}."up" ("mouse type") -> [_ w391 w404]
          frame "normal", Default {
          }
          frame "select noise" {
            n179 = call "_PC_Spectrafilter enable_draw_rectangle.vi"("error in (no error)"=w392, "mouse type"=w391, "Point32"=w389, "xy graph ref"=w390) -> ("error out"=w386:errorcluster, "max value"=w387:dbl, "min value"=w388:dbl)  [unwired: 5 in]
            n180 = Bundle By Name(cluster=cluster{"noise start":dbl, "noise end":dbl} {"noise start"=0.0, "noise end"=0.0}, "noise start"=w388, "noise end"=w387) -> (w393:cluster{"noise start":dbl, "noise end":dbl})
            n181 = call "_QMH_Enqueue.vi"("error in (no error)"=w386, "Data"=w393, "Msg"="SaveProcess", "QMH in"=w395) -> ()  [unwired: 6 in, 2 out]
          }
          frame "select signal" {
            n182 = call "_PC_Spectrafilter enable_draw_rectangle.vi"("error in (no error)"=w405, "mouse type"=w404, "Point32"=w402, "xy graph ref"=w403) -> ("error out"=w401:errorcluster, "max value"=w398:dbl, "min value"=w399:dbl)  [unwired: 5 in]
            n183 = Bundle By Name(cluster=cluster{"signal start":dbl, "signal end":dbl} {"signal start"=0.0, "signal end"=0.0}, "signal start"=w399, "signal end"=w398) -> (w397:cluster{"signal start":dbl, "signal end":dbl})
            n184 = call "_QMH_Enqueue.vi"("error in (no error)"=w401, "Data"=w397, "Msg"="SaveProcess", "QMH in"=w406) -> ()  [unwired: 6 in, 2 out]
          }
        }
      }
      event "Cursor": Value Change {
        n185 = event-data() -> ("NewVal"=w408:bool)  [unwired: 1 in]
        n186 = control-ref of="XY Graph"() -> (w412:refnum<vi>)
        n187 = property class="XYGraph (strict)"(reference=w412, "Active Cursor"=u32 0) -> (reference out=w410:refnum<vi>, error out=w409:errorcluster)  [unwired: 1 in]
        n188 = property class="XYGraph (strict)"(reference=w410, error in=w409, "Cursor.Visible"=w408) -> ()  [unwired: 2 out]
      }
      event "timeDomain": Value Change {
        n189 = event-data() -> ()  [unwired: 1 in, 1 out]
        n190 = call "_QMH_Enqueue.vi"("error in (no error)"=w414, "Msg"="updSpecGraph", "QMH in"=w415) -> ()  [unwired: 7 in, 2 out]
      }
      event "SigProc.Enable": Value Change {
        n191 = event-data() -> ("NewVal"=w423:bool)  [unwired: 1 in]
        n192 = call <vilib>:"Set Busy.vi"("error in (no error)"=w422) -> ("error out"=w421:errorcluster)  [unwired: 9 in, 1 out]
        n193 = case shown="True" w423 {
          tunnel: [_ w430] -> w425
          tunnel: [w427 w429] -> w424
          tunnel: w421 -> [w427 w428]
          frame False {
          }
          frame True {
            n194 = call "SigProc_method pyProcess.vi"("func"=T14."loadScript", "error in (no error)"=w428) -> ("error out"=w429:errorcluster, "pyCode"=w430:string)  [unwired: 6 in, 2 out]
          }
        }
        n195 = call "SigProc_method pyProcess.vi"("replace?(T)"=FALSE, "func"=T14."newScript", "error in (no error)"=w424, "newScriptCode"=w425) -> ("error out"=w418:errorcluster)  [unwired: 4 in, 3 out]
        n196 = call "_QMH_Enqueue.vi"("error in (no error)"=w418, "Msg"="updSpecGraph", "QMH in"=w419) -> ("error out"=w417:errorcluster)  [unwired: 7 in, 1 out]
        n197 = call <vilib>:"Unset Busy.vi"("error in (no error)"=w417) -> ()  [unwired: 10 in, 1 out]
      }
      event "SigProc.Edit": Mouse Down {
        n198 = event-data() -> ()  [unwired: 1 in, 1 out]
        n199 = call "SigProc_method pyProcess.vi"("func"=T14."loadScript", "error in (no error)"=w438) -> ("error out"=w437:errorcluster, "pyCode"=w434:string)  [unwired: 6 in, 2 out]
        n200 = call "Sig2MS dialogPyScript.vi"("error in (no error)"=w437) -> ("error out"=w436:errorcluster)  [unwired: 10 in]
        n201 = call "SigProc_method pyProcess.vi"("func"=T14."loadScript", "error in (no error)"=w436) -> ("error out"=w432:errorcluster, "pyCode"=w435:string)  [unwired: 6 in, 2 out]
        n202 = Not Equal?(x=w434, y=w435) -> (x != y?=w433:bool)
        n203 = case shown="True" w433 {
          tunnel: w441 -> [_ w444]
          tunnel: w432 -> [_ w442]
          frame False {
          }
          frame True {
            n204 = call "_QMH_Enqueue.vi"("error in (no error)"=w442, "Msg"="updSpecGraph", "QMH in"=w444) -> ()  [unwired: 7 in, 2 out]
          }
        }
      }
      event "MergePlots": Value Change {
        n205 = event-data() -> ()  [unwired: 1 in, 1 out]
        n206 = call "_QMH_Enqueue.vi"("error in (no error)"=w445, "Msg"="mergeWfms", "QMH in"=w446) -> ()  [unwired: 7 in, 2 out]
      }
      event "listDataInfo": Mouse Down {
        n207 = event-data() -> ("CtlRef"=w450:refnum<vi>, "Mods.Double Click"=w448:bool)  [unwired: 1 in]
        n208 = case shown="False" w448 {
          tunnel: w450 -> [_ w458]
          tunnel: w449 -> [_ w457]
          frame False {
          }
          frame True {
            n209 = property class="MCListbox (strict)"(reference=w458, error in=w457) -> (reference out=w456:refnum<vi>, error out=w455:errorcluster, "Value"=w453:i32)
            n210 = Bundle By Name(cluster=T15 {"Row"=0, "Column"=0} ("Edit Position"), "Row"=w453, "Column"=2) -> (w452:T15)
            n211 = property class="MCListbox (strict)"(reference=w456, error in=w455, "EditPos"=w452) -> ()  [unwired: 2 out]
          }
        }
      }
      event "listDataInfo": Shortcut Menu Selection (User) {
        n212 = event-data() -> ("CtlRef"=w462:refnum<vi>, "ItemTag"=w461:string)  [unwired: 1 in]
        n213 = case shown="\"editRemark\"" w461 {
          tunnel: w462 -> [_ w471]
          tunnel: w460 -> [_ w470]
          tunnel: w459 -> [_ _]
          frame "False", Default {
          }
          frame "editRemark" {
            n214 = property class="MCListbox (strict)"(reference=w471, error in=w470, "Key Focus"=TRUE) -> (reference out=w469:refnum<vi>, error out=w468:errorcluster, "Value"=w466:i32)
            n215 = Bundle By Name(cluster=T15 {"Row"=0, "Column"=0} ("Edit Position"), "Row"=w466, "Column"=2) -> (w465:T15)
            n216 = property class="MCListbox (strict)"(reference=w469, error in=w468, "EditPos"=w465) -> ()  [unwired: 2 out]
          }
        }
      }
      event "listDataInfo": Edit Cell {
        n217 = event-data() -> ("CtlRef"=w483:refnum<vi>)  [unwired: 1 in]
        n218 = control-ref of="Item Names"() -> (w482:refnum<vi>)
        n219 = property class="Arr (strict)"(reference=w482, error in=w472) -> (reference out=w481:refnum<vi>, "Value"=w479:string[])  [unwired: 1 out]
        n220 = property class="MCListbox (strict)"(reference=w483, error in=w472) -> ("ItemNames"=w474:string[][])  [unwired: 2 out]
        n221 = Index Array(array=w474, index (col)=2 ("disabled index (col)")) -> (element=w477:string[])  [unwired: 1 in]
        n222 = Equal?(x=w479, y=w477) -> (x = y?=w476:bool[])
        n223 = Search 1D Array(1D array=w476, element=FALSE) -> (index of element=w475:i32)  [unwired: 1 in]
        n224 = case shown="0, Default" w475 {
          selector: w475 -> [w486 _]
          tunnel: w477 -> [w491 _]
          tunnel: w481 -> [w492 _]
          tunnel: w480 -> [w489 _]
          tunnel: w472 -> [w488 _]
          tunnel: w474 -> [w485 _]
          frame 0, Default {
            n225 = property class="Arr (strict)"(reference=w492, error in=w488, "Value"=w491) -> (error out=w487:errorcluster)  [unwired: 1 out]
            n226 = Index Array(array=w485, index (row)=w486) -> (element=w484:string[])  [unwired: 1 in]
            n227 = call "_QMH_Enqueue.vi"("error in (no error)"=w487, "Data"=w484, "Msg"="updListData", "QMH in"=w489) -> ()  [unwired: 6 in, 2 out]
          }
          frame -1 {
          }
        }
      }
      event "Document Path": Value Change {
        n228 = event-data() -> ("CtlRef"=w496:refnum<vi>, "OldVal"=w497:path, "NewVal"=w498:path)  [unwired: 1 in]
        n229 = Empty String/Path?(string/path=w498) -> (empty?=w501:bool)
        n230 = call <vilib>:"Check if File or Folder Exists.vi"("path"=w498) -> ("file or folder exists?"=w502:bool)  [unwired: 8 in, 2 out]
        n231 = Not(x=w501) -> (.not. x?=w500:bool)
        n232 = And(x=w500, y=w502) -> (x .and. y?=w499:bool)
        n233 = Select(t=w498, s=w499, f=w497) -> (s? t:f=w495:path)
        n234 = property class="Path"(reference=w496, error in=w494, "Value"=w495) -> (error out=w493:errorcluster)  [unwired: 1 out]
        n235 = call "_QMH_Enqueue.vi"("error in (no error)"=w493, "Msg"="updDocTree", "QMH in"=w504) -> ()  [unwired: 7 in, 2 out]
      }
      event "Undo": Value Change {
        n236 = event-data() -> ()  [unwired: 1 in, 1 out]
        n237 = control-ref of="Document Path"() -> (w509:refnum<vi>)
        n238 = property class="Path"(reference=w509) -> (reference out=w508:refnum<vi>, error out=w507:errorcluster, "Value"=w505:path)  [unwired: 1 in]
        n239 = Strip Path(path=w505) -> (stripped path=w506:path)  [unwired: 1 out]
        n240 = property class="Path"(reference=w508, error in=w507, "Val(Sgnl)"=w506) -> ()  [unwired: 2 out]
      }
      event "Document Tree": Shortcut Menu Activation? {
        n241 = event-data() -> ("MenuRef"=w514:refnum<k9>)  [unwired: 1 in]
        n242 = Delete Menu Items(9:w514) -> (0:w512:errorcluster, 3:w513:refnum<k9>)  [unwired: 3 in]
        n243 = Insert Menu Items(6:w512, 7:string[] ["Mount", "Rename", "SavaAs", "APP_SEPARATOR", "Delete"], 8:string[] ["Mount", "Rename", "SavaAs", "-", "Delete"], 9:w513) -> ()  [unwired: 2 in, 3 out]
        n244 = event-data("Discard?"=FALSE) -> ()  [unwired: 1 in, 1 out]
      }
      event "Document Tree": Double Click {
        n245 = event-data() -> ("CtlRef"=w524:refnum<vi>, "Tag"=w522:string)  [unwired: 1 in]
        n246 = property class="Tree (strict)"(reference=w524, error in=w521, "Active Item Tag"=w522) -> (reference out=w525:refnum<vi>, error out=w520:errorcluster)
        n247 = property class="Tree (strict)"(reference=w525, error in=w520) -> (error out=w519:errorcluster, "Glyph"=w523:i32)  [unwired: 1 out]
        n248 = String To Path(string=w522) -> (path=w517:path)
        n249 = case shown="13" w523 {
          tunnel: w519 -> [_ w526 w531]
          tunnel: w518 -> [_ w528 _]
          tunnel: w517 -> [_ w527 w530]
          tunnel: w516 -> [_ _ w532]
          frame 0, Default {
          }
          frame 13 {
            n250 = call "_QMH_Enqueue.vi"("error in (no error)"=w526, "Data"=w527, "Msg"="updFileTree", "QMH in"=w528) -> ()  [unwired: 6 in, 2 out]
          }
          frame 14 {
            n251 = property class="Path"(reference=w532, error in=w531, "Val(Sgnl)"=w530) -> ()  [unwired: 2 out]
          }
        }
      }
      event "Document Tree": Shortcut Menu Selection (User) {
        n252 = event-data() -> ("ItemTag"=w533:string, "CtlRef"=w537:refnum<vi>, "Coords"=w536:T17)  [unwired: 1 in]
        n253 = case shown="Default" w533 {
          selector: w533 -> [_ _ _ w579]
          tunnel: w537 -> [w542 w562 _ w583]
          tunnel: w536 -> [_ _ _ w582]
          tunnel: w535 -> [w540 w558 w574 w581]
          tunnel: w534 -> [w539 w557 w573 w580]
          frame "Mount" {
            n254 = property class="Tree (strict)"(reference=w542) -> (reference out=w541:refnum<vi>, "Value"=w538:string[])  [unwired: 1 in, 1 out]
            n255 = for {
              tunnel: w541 -> [w547]
              tunnel: w540 -> [w546]
              tunnel: w539 -> [w545]
              tunnel: w538 -> [w544] mode=indexing
              n256 = property class="Tree (strict)"(reference=w547, "Active Item Tag"=w544) -> (reference out=w548:refnum<vi>)  [unwired: 1 in, 1 out]
              n257 = property class="Tree (strict)"(reference=w548) -> ("Glyph"=w543:i32)  [unwired: 1 in, 2 out]
              n258 = case shown="13" w543 {
                tunnel: w546 -> [_ w552]
                tunnel: w545 -> [_ w551]
                tunnel: w544 -> [_ w550]
                frame 0, Default {
                }
                frame 13 {
                  n259 = String To Path(string=w550) -> (path=w553:path)
                  n260 = call "_QMH_Enqueue.vi"("error in (no error)"=w551, "Data"=w553, "Msg"="updFileTree", "QMH in"=w552) -> ()  [unwired: 6 in, 2 out]
                }
              }
            }
          }
          frame "MergeGroup" {
            n261 = property class="Tree (strict)"(reference=w562) -> (reference out=w561:refnum<vi>, "Value"=w554:string[])  [unwired: 1 in, 1 out]
            n262 = for {
              tunnel: w561 -> [w567]
              tunnel: w554 -> [w564] mode=indexing
              shift-right: [w563] -> w556
              shift-left: string[] [] -> [w565]
              n263 = property class="Tree (strict)"(reference=w567, "Active Item Tag"=w564) -> (reference out=w568:refnum<vi>)  [unwired: 1 in, 1 out]
              n264 = property class="Tree (strict)"(reference=w568) -> ("Glyph"=w566:i32)  [unwired: 1 in, 2 out]
              n265 = case shown="13" w566 {
                tunnel: w565 -> [w569 w572]
                tunnel: [w569 w570] -> w563
                tunnel: w564 -> [_ w571]
                frame 0, Default {
                }
                frame 13 {
                  n266 = Build Array (concatenate)(w572, w571) -> (w570:string[])
                }
              }
            }
            n267 = String To Path(string=w556) -> (path=w555:path[])
            n268 = call "_QMH_Enqueue.vi"("error in (no error)"=w557, "Data"=w555, "Msg"="MergeGroup", "QMH in"=w558) -> ()  [unwired: 6 in, 2 out]
          }
          frame "Save As" {
            n269 = call "_QMH_Enqueue.vi"("error in (no error)"=w573, "Msg"="moveFile", "QMH in"=w574) -> ()  [unwired: 7 in, 2 out]
          }
          frame Default {
            n270 = invoke class="Tree (strict)" method="Point To Row Column"(reference=w583, "Point"=w582) -> ("Tag"=w584:string)  [unwired: 6 in, 7 out]
            n271 = case shown="\"Delete\"" w579 {
              tunnel: [_ "deleteFile"] -> w585
              frame "None", Default {
              }
              frame "Delete" {
              }
            }
            n272 = call "_QMH_Enqueue.vi"("error in (no error)"=w580, "Data"=w584, "Msg"=w585, "QMH in"=w581) -> ("error out"=w577:errorcluster, "QMH out"=w578:refnum<class "QMH.lvclass">)  [unwired: 6 in]
            n273 = call "_QMH_Enqueue.vi"("error in (no error)"=w577, "Msg"="updDocTree", "QMH in"=w578) -> ()  [unwired: 7 in, 2 out]
          }
        }
      }
      event "File Tree": Value Change {
        n274 = event-data() -> ("CtlRef"=w588:refnum<vi>, "NewVal"=w587:string[])  [unwired: 1 in]
        n275 = Array Size(array=w587) -> (size(s)=w595:i32)
        n276 = Greater?(x=w595, y=1) -> (0:w593:bool)
        n277 = case shown="True" w593 {
          tunnel: w588 -> [w596 w603]
          tunnel: w587 -> [w597 w602]
          tunnel: string[] [] ("NewVal") -> [_ w601]
          tunnel: [w596 w600] -> w591
          tunnel: [_ w599] -> w590
          tunnel: [w597 w598] -> w589
          frame False {
          }
          frame True {
            n278 = for {
              tunnel: w602 -> [w612] mode=indexing
              shift-right: [w607] -> w598
              shift-left: w601 -> [w608]
              shift-right: [w606] -> w600
              shift-left: w603 -> [w615]
              shift-right: [w604] -> w599
              shift-left: _ -> [w605]
              n279 = property class="Tree (strict)"(reference=w615, error in=w605, "Active Item Tag"=w612) -> (reference out=w614:refnum<vi>, error out=w613:errorcluster)
              n280 = property class="Tree (strict)"(reference=w614, error in=w613) -> (reference out=w606:refnum<vi>, error out=w604:errorcluster, "Indent Level"=w611:i32)
              n281 = Build Array (concatenate)(w608, w612) -> (w609:string[])
              n282 = Equal To 0?(x=w611) -> (x = 0?=w610:bool)
              n283 = Select(t=w608, s=w610, f=w609) -> (s? t:f=w607:string[])
            }
          }
        }
        n284 = property class="Tree (strict)"(reference=w591, error in=w590, "Value"=w589) -> ()  [unwired: 2 out]
      }
      event "File Tree": Shortcut Menu Activation? {
        n285 = event-data() -> ("CtlRef"=w618:refnum<vi>, "MenuRef"=w617:refnum<k9>)  [unwired: 1 in]
        n286 = call "DataTreeCtrl setFileTreeMenu.vi"("error in (no error)"=w616, "menuRefnum"=w617, "fileTreeRefnum"=w618) -> ()  [unwired: 8 in, 1 out]
        n287 = event-data("Discard?"=FALSE) -> ()  [unwired: 1 in, 1 out]
      }
      event "File Tree": Key Down; "File Tree": Key Repeat {
        n288 = event-data() -> ("CtlRef"=w620:refnum<vi>, "VKey"=w623:T16)  [unwired: 1 in]
        n289 = case shown="\"Up\"" w623 {
          tunnel: w622 -> [_ w626 w641]
          tunnel: w621 -> [_ w625 w640]
          tunnel: w620 -> [_ w632 w647]
          frame "ASCII", Default {
          }
          frame "Down" {
            n290 = property class="Tree (strict)"(reference=w632) -> (reference out=w629:refnum<vi>, "Value"=w631:string[])  [unwired: 1 in, 1 out]
            n291 = Index Array(array=w631, index=0) -> (element=w624:string)
            n292 = property class="Tree (strict)"(reference=w629, "Active Item Tag"=w624) -> (reference out=w633:refnum<vi>)  [unwired: 1 in, 1 out]
            n293 = property class="Tree (strict)"(reference=w633) -> ("Indent Level"=w628:i32)  [unwired: 1 in, 2 out]
            n294 = Equal To 0?(x=w628) -> (x = 0?=w627:bool)
            n295 = case shown="True" w627 {
              tunnel: w626 -> [w638 _]
              tunnel: w625 -> [w637 _]
              tunnel: w624 -> [w634 _]
              frame False {
                n296 = String To Path(string=w634) -> (path=w635:path)
                n297 = call "_QMH_Enqueue.vi"("error in (no error)"=w637, "Data"=w635, "Msg"="updSpecGraph", "QMH in"=w638) -> ()  [unwired: 6 in, 2 out]
              }
              frame True {
              }
            }
          }
          frame "Up" {
            n298 = property class="Tree (strict)"(reference=w647) -> (reference out=w644:refnum<vi>, "Value"=w646:string[])  [unwired: 1 in, 1 out]
            n299 = Index Array(array=w646, index=0) -> (element=w639:string)
            n300 = property class="Tree (strict)"(reference=w644, "Active Item Tag"=w639) -> (reference out=w648:refnum<vi>)  [unwired: 1 in, 1 out]
            n301 = property class="Tree (strict)"(reference=w648) -> ("Indent Level"=w643:i32)  [unwired: 1 in, 2 out]
            n302 = Equal To 0?(x=w643) -> (x = 0?=w642:bool)
            n303 = case shown="False" w642 {
              tunnel: w641 -> [w653 _]
              tunnel: w640 -> [w652 _]
              tunnel: w639 -> [w649 _]
              frame False {
                n304 = String To Path(string=w649) -> (path=w650:path)
                n305 = call "_QMH_Enqueue.vi"("error in (no error)"=w652, "Data"=w650, "Msg"="updSpecGraph", "QMH in"=w653) -> ()  [unwired: 6 in, 2 out]
              }
              frame True {
              }
            }
          }
        }
      }
      event "File Tree": Double Click {
        n306 = event-data() -> ("CtlRef"=w658:refnum<vi>, "Tag"=w657:string)  [unwired: 1 in]
        n307 = property class="Tree (strict)"(reference=w658, "Active Item Tag"=w657) -> (reference out=w656:refnum<vi>)  [unwired: 1 in, 1 out]
        n308 = property class="Tree (strict)"(reference=w656) -> ("Indent Level"=w655:i32)  [unwired: 1 in, 2 out]
        n309 = Equal To 0?(x=w655) -> (x = 0?=w654:bool)
        n310 = case shown="False" w654 {
          tunnel: w660 -> [w665 _]
          tunnel: w659 -> [w664 _]
          tunnel: w657 -> [w661 _]
          frame False {
            n311 = String To Path(string=w661) -> (path=w662:path)
            n312 = call "_QMH_Enqueue.vi"("error in (no error)"=w664, "Data"=w662, "Msg"="updSpecGraph", "QMH in"=w665) -> ()  [unwired: 6 in, 2 out]
          }
          frame True {
          }
        }
      }
      event "File Tree": Shortcut Menu Selection (User) {
        n313 = event-data() -> ("CtlRef"=w668:refnum<vi>, "Coords"=w667:T17, "ItemTag"=w666:string)  [unwired: 1 in]
        n314 = case shown="\"delete\"" w666 {
          selector: w666 -> [w671 _]
          tunnel: w670 -> [w677 w687]
          tunnel: w669 -> [w676 w686]
          tunnel: w668 -> [w675 w689]
          tunnel: w667 -> [w674 _]
          frame "else", Default {
            n315 = case shown="\"saveAsMAT\"" w671 {
              tunnel: [_ "unmount" "updSpecGraph" "updIonGraph" "loadScript" "loadInstr" "saveAsMAT"] -> w673
              frame "None", Default {
              }
              frame "unmount" {
              }
              frame "loadData" {
              }
              frame "loadIonisation" {
              }
              frame "loadScript" {
              }
              frame "loadInstrument" {
              }
              frame "saveAsMAT" {
              }
            }
            n316 = invoke class="Tree (strict)" method="Point To Row Column"(reference=w675, "Point"=w674) -> ("Tag"=w672:string)  [unwired: 6 in, 7 out]
            n317 = call "_QMH_Enqueue.vi"("error in (no error)"=w676, "Data"=w672, "Msg"=w673, "QMH in"=w677) -> ()  [unwired: 6 in, 2 out]
          }
          frame "delete" {
            n318 = property class="Tree (strict)"(reference=w689) -> (reference out=w685:refnum<vi>, error out=w684:errorcluster, "Indent Level"=w688:i32)  [unwired: 1 in]
            n319 = case shown="0" w688 {
              tunnel: w687 -> [_ w701 w703]
              tunnel: w686 -> [_ w690 w702]
              tunnel: w685 -> [_ w699 _]
              tunnel: w684 -> [_ w698 _]
              frame -1, Default {
              }
              frame 0 {
                n320 = property class="Tree (strict)"(reference=w699, error in=w698) -> ("Value"=w694:string[])  [unwired: 2 out]
                n321 = Index Array(array=w694, index=0) -> (element=w692:string)
                n322 = String To Path(string=w692) -> (path=w691:path)
                n323 = call "_QMH_Enqueue.vi"("error in (no error)"=w690, "Data"=w691, "Msg"="deleteCustomFile", "QMH in"=w701) -> ("error out"=w696:errorcluster, "QMH out"=w697:refnum<class "QMH.lvclass">)  [unwired: 6 in]
                n324 = call "_QMH_Enqueue.vi"("error in (no error)"=w696, "Msg"="updDocTree", "QMH in"=w697) -> ()  [unwired: 7 in, 2 out]
              }
              frame 1 {
                n325 = call "_QMH_Enqueue.vi"("error in (no error)"=w702, "Msg"="deleteData", "QMH in"=w703) -> ()  [unwired: 7 in, 2 out]
              }
            }
          }
        }
      }
      event "File Tree": Drag Starting? {
        n326 = event-data() -> ("CtlRef"=w708:refnum<vi>)  [unwired: 1 in]
        n327 = property class="Tree (strict)"(reference=w708) -> (reference out=w706:refnum<vi>, "Value"=w707:string[])  [unwired: 1 in, 1 out]
        n328 = for {
          tunnel: w707 -> [w712] mode=indexing
          tunnel: w706 -> [w713]
          tunnel: [w709] -> w705
          stop <- w709 stop-if-true
          n329 = property class="Tree (strict)"(reference=w713, "Active Item Tag"=w712) -> (reference out=w711:refnum<vi>)  [unwired: 1 in, 1 out]
          n330 = property class="Tree (strict)"(reference=w711) -> ("Indent Level"=w710:i32)  [unwired: 1 in, 2 out]
          n331 = Equal To 0?(x=w710) -> (x = 0?=w709:bool)
        }
        n332 = event-data("Discard?"=w705) -> ()  [unwired: 1 in, 1 out]
      }
      event "File Tree": Drop {
        n333 = event-data() -> ("CtlRef"=w727:refnum<vi>, "Coords"=w731:T17)  [unwired: 1 in]
        n334 = invoke class="Tree (strict)" method="Point To Row Column"(reference=w727, "Point"=w731) -> (reference out=w722:refnum<vi>, error out=w721:errorcluster, "Tag"=w720:string)  [unwired: 6 in, 5 out]
        n335 = invoke class="Tree (strict)" method="Navigate Tree.Get Parent"(reference=w722, error in=w721, "tag"=w720) -> (error out=w717:errorcluster, "Navigate Tree:Get Parent"=w726:string)  [unwired: 1 in, 2 out]
        n336 = Empty String/Path?(string/path=w726) -> (empty?=w725:bool)
        n337 = property class="Tree (strict)"(reference=w727, error in=w717) -> (error out=w716:errorcluster, "Value"=w723:string[])  [unwired: 1 out]
        n338 = Select(t=w720, s=w725, f=w726) -> (s? t:f=w718:string)
        n339 = Empty String/Path?(string/path=w718) -> (empty?=w715:bool)
        n340 = Or(x=w716, y=w715) -> (x .or. y?=w714:bool)
        n341 = Bundle By Name(cluster=T7 {"selectDataArr"=[], "tagFilePath"=""}, "selectDataArr"=w723, "tagFilePath"=w718) -> (w719:T7)
        n342 = case shown="False" w714 {
          tunnel: w730 -> [w735 _]
          tunnel: w729 -> [w734 _]
          tunnel: w719 -> [w733 _]
          frame False {
            n343 = call "_QMH_Enqueue.vi"("error in (no error)"=w734, "Data"=w733, "Msg"="moveData", "QMH in"=w735) -> ()  [unwired: 6 in, 2 out]
          }
          frame True {
          }
        }
        n344 = event-data("Accepted?"=FALSE) -> ()  [unwired: 1 in, 1 out]
      }
      event Panel Close {
        n345 = event-data() -> ()  [unwired: 1 in, 4 out]
        n346 = call "_QMH_Enqueue.vi"("error in (no error)"=w737, "Msg"="close", "QMH in"=w738) -> ()  [unwired: 7 in, 2 out]
      }
      event Key Down? {
        n347 = event-data() -> ("VKey"=w742:T16)  [unwired: 1 in]
        n348 = Equal?(x=w742, y=eventvkey."Escape") -> (x = y?=w740:bool)
        n349 = case shown="True" w740 {
          tunnel: w744 -> [_ w746]
          tunnel: w743 -> [_ w745]
          frame False {
          }
          frame True {
            n350 = call "_QMH_Enqueue.vi"("error in (no error)"=w745, "Msg"="Exit", "QMH in"=w746) -> ()  [unwired: 7 in, 2 out]
          }
        }
        n351 = event-data("Discard?"=w740) -> ()  [unwired: 1 in, 1 out]
      }
    }
  }
  n352 = call <vilib>:"Clear Errors.vi"("error in (no error)"=w36) -> ("error out"=→"error out":errorcluster)  [unwired: 5 in, 1 out]
